vi "STARTFIXWAVEFORM2.vi"() -> ()   [LabVIEW 2024]
uses:
  <vilib>/Utility/file.llb/Read Delimited Spreadsheet (DBL).vi
panel:
  in  "Flow Rate Lower Limit 2":dbl
  in  "Flow Rate Upper Limit 2":dbl
  in  "Desired Flow Rate 3":dbl format="%_2f"
  in  "Initial RPM  3":dbl format="%_4f"
  in  "stop 2":bool
  out "Boolean":bool
  out "Waveform Chart 3":dbl[](graph)
  out "Waveform Chart 2":dbl(graph)
  out "Flow Rate":dbl(graph)
  in  "Color Box":u32(colorbox)
  # "Blood Flow Rate"
  # "Flow Rate (mL/min)"
  # "Initial LVAD Speed (RPM)"
  # "Desired Flow Rate (mL/min)"
  # "LVAD Speed"
  # "Upper Flow Rate Limit (mL/min)"
  # "Speed (RPM)"
  # "Lower Flow Rate Limit (mL/min)"
  # "Optimal Flow State"
  # "Right Heart Waveform"
  # "Amplitude"
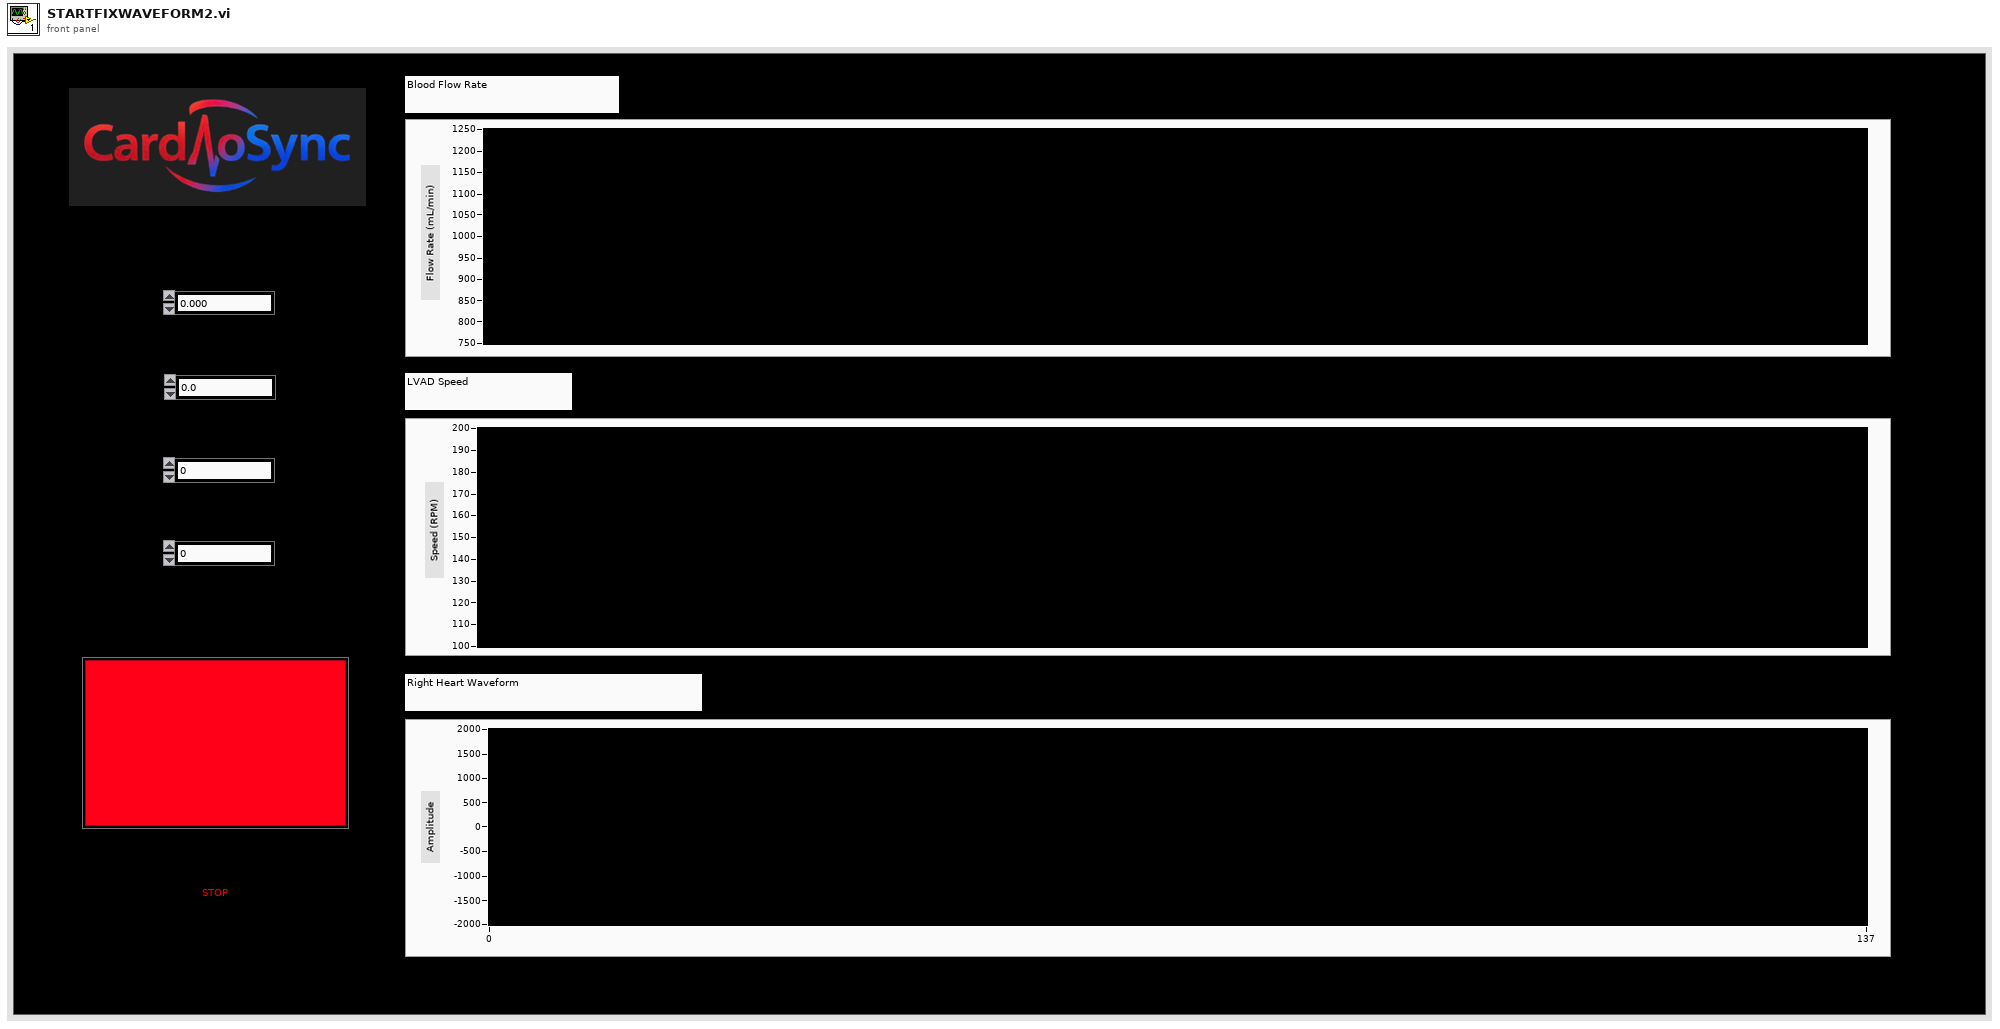
[diagram p1: front panel]
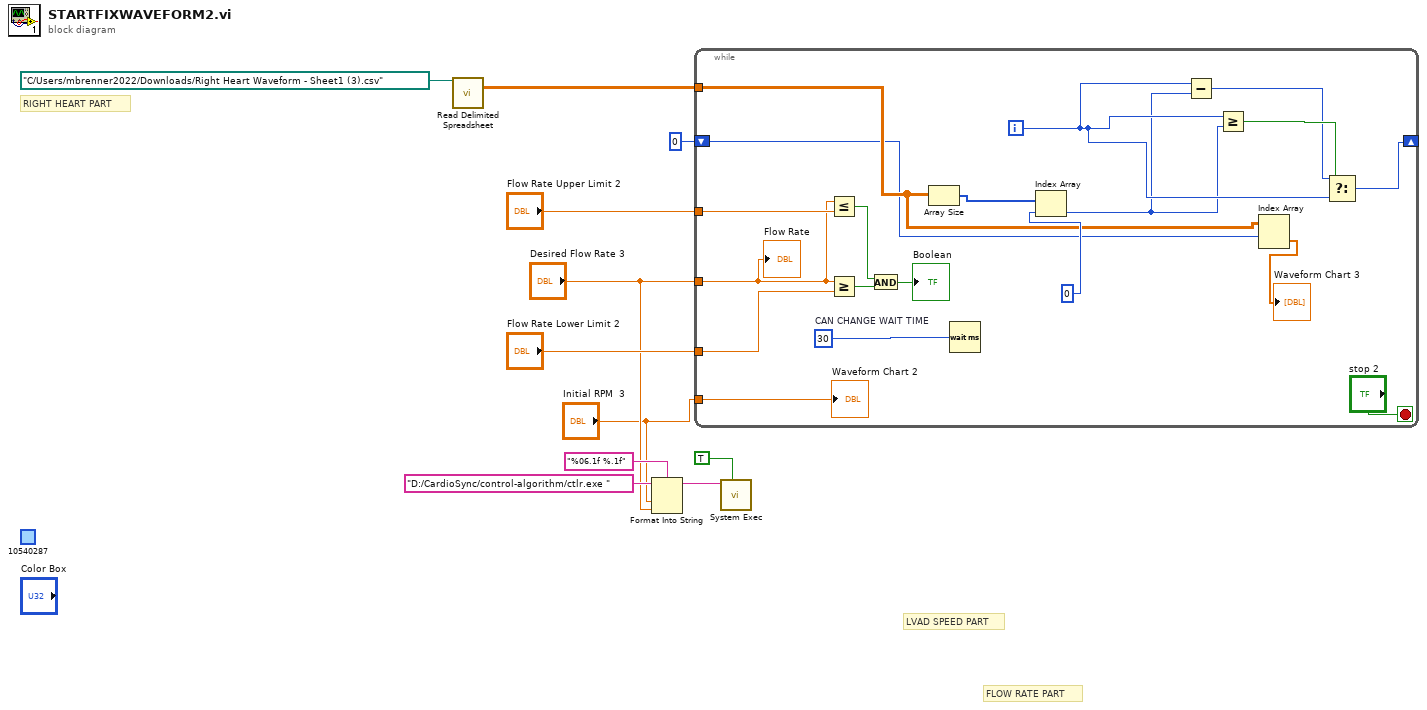
[diagram p0: block diagram]
diagram:
  (unwired) u32 10540287 ("Color Box 2")
  # "FLOW RATE PART"
  # "LVAD SPEED PART"
  # "RIGHT HEART PART"
  n1 = call-poly <vilib>:"Read Delimited Spreadsheet.vi"("file path (dialog if empty)"=path "C:/Users/mbrenner2022/Downloads/Right Heart Waveform - Sheet1 (3).csv") -> ("all rows"=w2:dbl[][])  [unwired: 9 in, 5 out]
  n2 = Format Into String(format string="%06.1f %.1f", initial string="D:/CardioSync/control-algorithm/ctlr.exe ", "Initial RPM  3", "Desired Flow Rate 3") -> (resulting string=w7:string)  [unwired: 1 in, 1 out]
  n3 = while {
    tunnel: "Flow Rate Upper Limit 2" -> [w26]
    tunnel: "Flow Rate Lower Limit 2" -> [w25]
    tunnel: "Desired Flow Rate 3" -> [w24]
    tunnel: "Initial RPM  3" -> [w23]
    tunnel: w2 -> [w19]
    shift-right: [w13] -> _
    shift-left: 0 -> [w18]
    i -> [w16]
    stop <- "stop 2" stop-if-true
    w30 = u32 30  # CAN CHANGE WAIT TIME
    n4 = Less Or Equal?(x=w24, y=w26) -> (x <= y?=w29:bool)
    n5 = Greater Or Equal?(x=w24, y=w25) -> (x >= y?=w28:bool)
    n6 = And(x=w29, y=w28) -> (x .and. y?=→"Boolean":bool)
    n7 = Array Size(array=w19) -> (size(s)=w21:i32[])
    n8 = Wait (ms)(milliseconds to wait=w30) -> ()  [unwired: 1 out]
    n9 = Index Array(array=w21, index=0) -> (element=w12:i32)
    n10 = Subtract(x=w16, y=w12) -> (x-y=w14:i32)
    n11 = Greater Or Equal?(x=w16, y=w12) -> (x >= y?=w15:bool)
    n12 = Index Array(array=w19, index (row)=w18) -> (element=→"Waveform Chart 3":dbl[])  [unwired: 1 in]
    n13 = Select(t=w14, s=w15, f=w16) -> (s? t:f=w13:i32)
    "Waveform Chart 2" <- w23
    "Flow Rate" <- w24
  }
  n14 = call <vilib>:"System Exec.vi"("wait until completion? (T)"=TRUE, "command line"=w7) -> ()  [unwired: 6 in, 4 out]
